vi "data_waypoint_ref.vi"() -> ()   [LabVIEW 2019] (continued)
"Y"=530152.5967771014}, {"X"=175289.23222510127, "Y"=530152.6409434144}, {"X"=175289.26360565764, "Y"=530152.6851751207}, {"X"=175289.29417483156, "Y"=530152.7294092241}, {"X"=175289.32498934455, "Y"=530152.7727347375}, {"X"=175289.35533826269, "Y"=530152.8164722754}, {"X"=175289.385890799, "Y"=530152.8604711375}, {"X"=175289.41661120942, "Y"=530152.904625996}, {"X"=175289.4478910891, "Y"=530152.9495616502}, {"X"=175289.47917020373, "Y"=530152.9951376967}, {"X"=175289.5106185431, "Y"=530153.0407265619}, {"X"=175289.54200313758, "Y"=530153.08602594}, {"X"=175289.5739645148, "Y"=530153.130472353}, {"X"=175289.60522496788, "Y"=530153.1748287205}, {"X"=175289.6366590831, "Y"=530153.2192023303}, {"X"=175289.6678968938, "Y"=530153.2639904988}, {"X"=175289.69931618578, "Y"=530153.3099423731}, {"X"=175289.73108270628, "Y"=530153.3561928844}, {"X"=175289.76287250203, "Y"=530153.402526566}, {"X"=175289.7944634813, "Y"=530153.4493247548}, {"X"=175289.82722049116, "Y"=530153.4953348278}, {"X"=175289.8601326513, "Y"=530153.5407928433}, {"X"=175289.89234136775, "Y"=530153.5862074348}, {"X"=175289.9231350958, "Y"=530153.6320945667}, {"X"=175289.95472487184, "Y"=530153.6784854437}, {"X"=175289.98763897427, "Y"=530153.7249001521}, {"X"=175290.0213877559, "Y"=530153.7711048503}, {"X"=175290.05441688612, "Y"=530153.8180774795}, {"X"=175290.0870279125, "Y"=530153.865045794}, {"X"=175290.1190894426, "Y"=530153.9119114052}, {"X"=175290.15082290868, "Y"=530153.9583695601}, {"X"=175290.18253651966, "Y"=530154.004402696}, {"X"=175290.215824471, "Y"=530154.0499339624}, {"X"=175290.24876343764, "Y"=530154.0957714727}, {"X"=175290.28090772417, "Y"=530154.1421662602}, {"X"=175290.31260737777, "Y"=530154.1888720124}, {"X"=175290.34510314872, "Y"=530154.2349083878}, {"X"=175290.37745346018, "Y"=530154.2805800489}, {"X"=175290.40967781737, "Y"=530154.3255950455}, {"X"=175290.4415173953, "Y"=530154.3698930992}, {"X"=175290.47334424395, "Y"=530154.4146795312}, {"X"=175290.50540644318, "Y"=530154.4602743543}, {"X"=175290.5380738031, "Y"=530154.5068251977}, {"X"=175290.57155401353, "Y"=530154.5544701797}, {"X"=175290.60687618723, "Y"=530154.6022528902}, {"X"=175290.64227715097, "Y"=530154.6503194917}, {"X"=175290.6771000642, "Y"=530154.6985121064}, {"X"=175290.71074572636, "Y"=530154.7463930005}, {"X"=175290.74366782108, "Y"=530154.7937166628}, {"X"=175290.77674741115, "Y"=530154.8397823889}, {"X"=175290.8104922183, "Y"=530154.8852446075}, {"X"=175290.84345047412, "Y"=530154.9319166768}, {"X"=175290.8771305831, "Y"=530154.9791648488}, {"X"=175290.91168912026, "Y"=530155.0269198505}, {"X"=175290.94661003543, "Y"=530155.0750045214}, {"X"=175290.981122192, "Y"=530155.1229516666}, {"X"=175291.01579159318, "Y"=530155.1701547412}, {"X"=175291.04955919375, "Y"=530155.2164370784}, {"X"=175291.08231414267, "Y"=530155.262653598}, {"X"=175291.11492730505, "Y"=530155.3085508951}, {"X"=175291.14872001382, "Y"=530155.3537377286}, {"X"=175291.182644366, "Y"=530155.3991095183}, {"X"=175291.21636701853, "Y"=530155.4442699214}, {"X"=175291.24936465317, "Y"=530155.4895811882}, {"X"=175291.28248111415, "Y"=530155.5349365}, {"X"=175291.31537208255, "Y"=530155.580122668}, {"X"=175291.348325878, "Y"=530155.6252864538}, {"X"=175291.38153227052, "Y"=530155.6705005467}, {"X"=175291.41516056712, "Y"=530155.7158055122}, {"X"=175291.44858402072, "Y"=530155.7616338248}, {"X"=175291.48274548614, "Y"=530155.8069127973}, {"X"=175291.51713847913, "Y"=530155.8517049672}, {"X"=175291.55134679007, "Y"=530155.8960504106}, {"X"=175291.58456519523, "Y"=530155.9396351947}, {"X"=175291.61696642355, "Y"=530155.9821591497}, {"X"=175291.6479902135, "Y"=530156.023771541}, {"X"=175291.6785537982, "Y"=530156.0649235916}, {"X"=175291.70969666803, "Y"=530156.1063669323}, {"X"=175291.7420121854, "Y"=530156.1480631868}, {"X"=175291.77421945485, "Y"=530156.1905977037}, {"X"=175291.80641845273, "Y"=530156.2342298953}, {"X"=175291.83880961206, "Y"=530156.2778426528}, {"X"=175291.8714862793, "Y"=530156.3212525729}, {"X"=175291.903615614, "Y"=530156.3652911794}, {"X"=175291.9363788722, "Y"=530156.4089272545}, {"X"=175291.9693198524, "Y"=530156.4530544727}, {"X"=175292.00263982284, "Y"=530156.4980373809}, {"X"=175292.03573972572, "Y"=530156.5440875158}, {"X"=175292.06968311957, "Y"=530156.5908099515}, {"X"=175292.10416577995, "Y"=530156.6374730819}, {"X"=175292.13854745447, "Y"=530156.6838335177}, {"X"=175292.1720661163, "Y"=530156.7301088271}, {"X"=175292.2050774269, "Y"=530156.7758551223}, {"X"=175292.23774666685, "Y"=530156.8212483841}, {"X"=175292.2703950841, "Y"=530156.8658914415}, {"X"=175292.30284617713, "Y"=530156.9103042324}, {"X"=175292.33573019976, "Y"=530156.9552418168}, {"X"=175292.3690841089, "Y"=530157.0006197365}, {"X"=175292.40287209605, "Y"=530157.0463115734}, {"X"=175292.43625491866, "Y"=530157.0924818472}, {"X"=175292.46991898818, "Y"=530157.1379065764}, {"X"=175292.50292587615, "Y"=530157.1830557807}, {"X"=175292.53606117488, "Y"=530157.2272967426}, {"X"=175292.56777705185, "Y"=530157.2717072674}, {"X"=175292.59928240773, "Y"=530157.317118397}, {"X"=175292.63191829307, "Y"=530157.3626160842}, {"X"=175292.66587593383, "Y"=530157.4075682566}, {"X"=175292.69985293486, "Y"=530157.4527767475}, {"X"=175292.73331970134, "Y"=530157.49827975}, {"X"=175292.76675738787, "Y"=530157.5444332153}, {"X"=175292.8009040642, "Y"=530157.5910063332}, {"X"=175292.8354354053, "Y"=530157.637958995}, {"X"=175292.87064782495, "Y"=530157.6854778919}, {"X"=175292.90666329346, "Y"=530157.7325748918}, {"X"=175292.94218916725, "Y"=530157.7803559012}, {"X"=175292.97651543948, "Y"=530157.8283546561}, {"X"=175293.01087843996, "Y"=530157.8758927135}, {"X"=175293.04497236086, "Y"=530157.9235003758}, {"X"=175293.07881658027, "Y"=530157.9705383087}, {"X"=175293.11260566092, "Y"=530158.0172023829}, {"X"=175293.14703717566, "Y"=530158.0636470264}, {"X"=175293.1813700373, "Y"=530158.1105791891}, {"X"=175293.21539555187, "Y"=530158.1584179054}, {"X"=175293.2495375595, "Y"=530158.205812335}, {"X"=175293.28470608912, "Y"=530158.252269229}, {"X"=175293.3199063943, "Y"=530158.2983886322}, {"X"=175293.35488698122, "Y"=530158.3438949328}, {"X"=175293.3886446154, "Y"=530158.389809945}, {"X"=175293.4223983855, "Y"=530158.4359169754}, {"X"=175293.45635716093, "Y"=530158.4824551338}, {"X"=175293.49104767398, "Y"=530158.5290177691}, {"X"=175293.52591940033, "Y"=530158.5751547926}, {"X"=175293.56061870293, "Y"=530158.6210958796}, {"X"=175293.59411550115, "Y"=530158.6668718222}, {"X"=175293.6271809516, "Y"=530158.7120597042}, {"X"=175293.65945930034, "Y"=530158.7576716585}, {"X"=175293.69267942, "Y"=530158.8030433188}, {"X"=175293.72706808845, "Y"=530158.8484792291}, {"X"=175293.76185547217, "Y"=530158.895451116}, {"X"=175293.7965144529, "Y"=530158.9433356876}, {"X"=175293.83203452808, "Y"=530158.9915551107}, {"X"=175293.86796527763, "Y"=530159.0399619979}, {"X"=175293.90361325, "Y"=530159.0885983519}, {"X"=175293.93887625565, "Y"=530159.1373534874}, {"X"=175293.97487363513, "Y"=530159.1852274456}, {"X"=175294.01073365632, "Y"=530159.2333814944}, {"X"=175294.04643691002, "Y"=530159.2821408798}, {"X"=175294.0818756446, "Y"=530159.3307123703}, {"X"=175294.11788264144, "Y"=530159.3791445598}, {"X"=175294.15405635608, "Y"=530159.4270401951}, {"X"=175294.19031250803, "Y"=530159.474657012}, {"X"=175294.2255617339, "Y"=530159.5217474012}, {"X"=175294.25969315338, "Y"=530159.5685591893}, {"X"=175294.29275883175, "Y"=530159.6156260639}, {"X"=175294.32651326683, "Y"=530159.6616609548}, {"X"=175294.3607518941, "Y"=530159.7075834295}, {"X"=175294.3953102612, "Y"=530159.754094294}, {"X"=175294.4301660572, "Y"=530159.800839571}, {"X"=175294.46538930168, "Y"=530159.8478312608}, {"X"=175294.5005892464, "Y"=530159.8944334593}, {"X"=175294.5360717114, "Y"=530159.9401191891}, {"X"=175294.57088286872, "Y"=530159.9855471951}, {"X"=175294.60512637242, "Y"=530160.0307227217}, {"X"=175294.63868134032, "Y"=530160.0764041571}, {"X"=175294.67373468378, "Y"=530160.1216560913}, {"X"=175294.7093190078, "Y"=530160.167040749}, {"X"=175294.74458629126, "Y"=530160.2136494077}, {"X"=175294.7794420138, "Y"=530160.2609707027}, {"X"=175294.81483305173, "Y"=530160.3092915086}, {"X"=175294.85090509735, "Y"=530160.3593561125}, {"X"=175294.88806120938, "Y"=530160.4102709948}, {"X"=175294.92585483048, "Y"=530160.4622982909}, {"X"=175294.96463635506, "Y"=530160.5147089018}, {"X"=175295.00314084318, "Y"=530160.5674932406}, {"X"=175295.04201721685, "Y"=530160.6190278914}, {"X"=175295.08002002342, "Y"=530160.6696039869}, {"X"=175295.1164572531, "Y"=530160.7191503169}, {"X"=175295.15120238528, "Y"=530160.7677160925}, {"X"=175295.18513989958, "Y"=530160.8154596288}, {"X"=175295.21911985, "Y"=530160.8622751979}, {"X"=175295.25361585215, "Y"=530160.908367834}, {"X"=175295.2882631498, "Y"=530160.9541026478}, {"X"=175295.3227068247, "Y"=530160.9995739195}, {"X"=175295.35650395526, "Y"=530161.0453733961}, {"X"=175295.39054459677, "Y"=530161.090246534}, {"X"=175295.4242712038, "Y"=530161.1346622286}, {"X"=175295.45741238436, "Y"=530161.1797045011}, {"X"=175295.49052893237, "Y"=530161.2251053321}, {"X"=175295.52422381577, "Y"=530161.2716753556}, {"X"=175295.5584969615, "Y"=530161.3190916035}, {"X"=175295.59356381797, "Y"=530161.3671225884}, {"X"=175295.62898613833, "Y"=530161.4158406355}, {"X"=175295.66490363725, "Y"=530161.4645672088}, {"X"=175295.70087106727, "Y"=530161.5140039441}, {"X"=175295.7368334574, "Y"=530161.563833585}, {"X"=175295.77286787695, "Y"=530161.6140581218}, {"X"=175295.80940447663, "Y"=530161.6645608615}, {"X"=175295.84631290415, "Y"=530161.7143954771}, {"X"=175295.88293148752, "Y"=530161.7641654665}, {"X"=175295.91866648968, "Y"=530161.8137837979}, {"X"=175295.95399056026, "Y"=530161.862829545}, {"X"=175295.9882959008, "Y"=530161.9112501208}, {"X"=175296.021704602, "Y"=530161.9589974427}, {"X"=175296.05467506434, "Y"=530162.0062210971}, {"X"=175296.08883693878, "Y"=530162.0522559017}, {"X"=175296.12335942886, "Y"=530162.0980232735}, {"X"=175296.15767913012, "Y"=530162.1438101135}, {"X"=175296.19184323237, "Y"=530162.18969841}, {"X"=175296.22616491732, "Y"=530162.2364574812}, {"X"=175296.26090724123, "Y"=530162.2837780067}, {"X"=175296.29650390253, "Y"=530162.3312458408}, {"X"=175296.33225156722, "Y"=530162.3800550482}, {"X"=175296.36839006183, "Y"=530162.4298308986}, {"X"=175296.40405752033, "Y"=530162.4808744899}, {"X"=175296.4404195736, "Y"=530162.5316652008}, {"X"=175296.4771856306, "Y"=530162.5818831403}, {"X"=175296.5143190418, "Y"=530162.6314185419}, {"X"=175296.55121999886, "Y"=530162.6796261277}, {"X"=175296.58696759774, "Y"=530162.7272156009}, {"X"=175296.62106253332, "Y"=530162.7745791067}, {"X"=175296.65513370547, "Y"=530162.8216951848}, {"X"=175296.6894842066, "Y"=530162.8689147633}, {"X"=175296.7245051825, "Y"=530162.9161112749}, {"X"=175296.7594826378, "Y"=530162.9641680548}, {"X"=175296.7949428259, "Y"=530163.0125164114}, {"X"=175296.83066872833, "Y"=530163.0611569866}, {"X"=175296.8668875833, "Y"=530163.1102511483}, {"X"=175296.90347265196, "Y"=530163.1594751914}, {"X"=175296.94033878695, "Y"=530163.2096906174}, {"X"=175296.97742890092, "Y"=530163.2601628694}, {"X"=175297.0145870955, "Y"=530163.3102930847}, {"X"=175297.0517672564, "Y"=530163.3603633035}, {"X"=175297.0892145761, "Y"=530163.4100154234}, {"X"=175297.1260384531, "Y"=530163.4594196689}, {"X"=175297.16179432158, "Y"=530163.5083098755}, {"X"=175297.1968335202, "Y"=530163.5568792308}, {"X"=175297.2321241116, "Y"=530163.6047908057}, {"X"=175297.26783519427, "Y"=530163.6517155846}, {"X"=175297.3031716078, "Y"=530163.6989466816}, {"X"=175297.3376430369, "Y"=530163.7460238435}, {"X"=175297.37241788793, "Y"=530163.7935651409}, {"X"=175297.40764496886, "Y"=530163.8421672372}, {"X"=175297.44412403886, "Y"=530163.8908943782}, {"X"=175297.4814756149, "Y"=530163.9405212577}, {"X"=175297.51936847973, "Y"=530163.9910710508}, {"X"=175297.5573672983, "Y"=530164.0433064074}, {"X"=175297.595877763, "Y"=530164.0960252604}, {"X"=175297.63482324645, "Y"=530164.1484764633}, {"X"=175297.67408375622, "Y"=530164.201420622}, {"X"=175297.71312810254, "Y"=530164.2540568792}, {"X"=175297.7516670672, "Y"=530164.3059288258}, {"X"=175297.78913671337, "Y"=530164.3565442422}, {"X"=175297.82573620637, "Y"=530164.4067560205}, {"X"=175297.8615577048, "Y"=530164.4559778853}, {"X"=175297.8972371134, "Y"=530164.5047762007}, {"X"=175297.93302551022, "Y"=530164.553887177}, {"X"=175297.96961301554, "Y"=530164.6033398478}, {"X"=175298.00658313325, "Y"=530164.653376285}, {"X"=175298.04413234367, "Y"=530164.7030403184}, {"X"=175298.08174063195, "Y"=530164.7529128302}, {"X"=175298.11949670635, "Y"=530164.8033376161}, {"X"=175298.15754264174, "Y"=530164.8535340244}, {"X"=175298.19573262517, "Y"=530164.9039153553}, {"X"=175298.2333517534, "Y"=530164.9547600736}, {"X"=175298.2709253971, "Y"=530165.0063984748}, {"X"=175298.30921058325, "Y"=530165.0575242384}, {"X"=175298.34725989297, "Y"=530165.108563021}, {"X"=175298.3849848592, "Y"=530165.160152141}, {"X"=175298.42313040857, "Y"=530165.2113859762}, {"X"=175298.46161175598, "Y"=530165.2629473361}, {"X"=175298.5006422235, "Y"=530165.3141863251}, {"X"=175298.53957860355, "Y"=530165.3662590976}, {"X"=175298.57924604914, "Y"=530165.4196282434}, {"X"=175298.61979824462, "Y"=530165.4744453614}, {"X"=175298.66179051698, "Y"=530165.5306877274}, {"X"=175298.70499840498, "Y"=530165.5885357952}, {"X"=175298.74955290352, "Y"=530165.6482533285}, {"X"=175298.79480152024, "Y"=530165.7087545921}, {"X"=175298.83997422215, "Y"=530165.7702460737}, {"X"=175298.8847225618, "Y"=530165.8314136203}, {"X"=175298.9291021474, "Y"=530165.8912926009}, {"X"=175298.97281817885, "Y"=530165.9496397171}, {"X"=175299.01543963805, "Y"=530166.0068768775}, {"X"=175299.05688362545, "Y"=530166.0634271845}, {"X"=175299.09825262203, "Y"=530166.1191808339}, {"X"=175299.13975714424, "Y"=530166.173434664}, {"X"=175299.18070865513, "Y"=530166.2269953544}, {"X"=175299.22062828136, "Y"=530166.2793770946}, {"X"=175299.25974002617, "Y"=530166.3308455878}, {"X"=175299.297952328, "Y"=530166.3812912287}, {"X"=175299.33612488734, "Y"=530166.4305771838}, {"X"=175299.37402761978, "Y"=530166.4784788326}, {"X"=175299.41189246927, "Y"=530166.5255504185}, {"X"=175299.44854593184, "Y"=530166.5730484385}, {"X"=175299.48464680242, "Y"=530166.620295045}, {"X"=175299.5206186963, "Y"=530166.667360014}, {"X"=175299.5570817157, "Y"=530166.7139596118}, {"X"=175299.59393444148, "Y"=530166.760246189}, {"X"=175299.63101704643, "Y"=530166.8075875615}, {"X"=175299.66873832993, "Y"=530166.8558371342}, {"X"=175299.70755977381, "Y"=530166.9049891003}, {"X"=175299.74702618556, "Y"=530166.954779551}, {"X"=175299.78702946118, "Y"=530167.0048947148}, {"X"=175299.8269780119, "Y"=530167.0550766316}, {"X"=175299.86691015412, "Y"=530167.1045016735}, {"X"=175299.9056200963, "Y"=530167.1539902581}, {"X"=175299.94444108658, "Y"=530167.202690514}, {"X"=175299.9832469312, "Y"=530167.2507615263}, {"X"=175300.02239172766, "Y"=530167.2984286564}, {"X"=175300.06160983795, "Y"=530167.3454263278}, {"X"=175300.10023907598, "Y"=530167.3924845605}, {"X"=175300.13795698716, "Y"=530167.4389938845}, {"X"=175300.17463229306, "Y"=530167.4854940797}, {"X"=175300.21027157555, "Y"=530167.53151233}, {"X"=175300.2456148467, "Y"=530167.5762784209}, {"X"=175300.28083256615, "Y"=530167.6208229107}, {"X"=175300.31683014592, "Y"=530167.6648911891}, {"X"=175300.35295156413, "Y"=530167.7092010507}, {"X"=175300.38885968522, "Y"=530167.754471571}, {"X"=175300.42531408952, "Y"=530167.7996572366}, {"X"=175300.4626722015, "Y"=530167.8446127126}, {"X"=175300.49978768127, "Y"=530167.8895922136}, {"X"=175300.5366776678, "Y"=530167.9350018955}, {"X"=175300.57296706524, "Y"=530167.9810026871}, {"X"=175300.60997343756, "Y"=530168.02653078}, {"X"=175300.64725950157, "Y"=530168.0722844577}, {"X"=175300.6848355032, "Y"=530168.1178341768}, {"X"=175300.72194708392, "Y"=530168.1629945957}, {"X"=175300.75843372697, "Y"=530168.2077007085}, {"X"=175300.79459920572, "Y"=530168.2516353095}, {"X"=175300.8309390622, "Y"=530168.2958279934}, {"X"=175300.86721646803, "Y"=530168.3407689049}, {"X"=175300.9041467231, "Y"=530168.3860186503}, {"X"=175300.94086441226, "Y"=530168.431876116}, {"X"=175300.97748970473, "Y"=530168.4773398549}, {"X"=175301.01311529457, "Y"=530168.5226245311}, {"X"=175301.04880451673, "Y"=530168.5675605212}, {"X"=175301.08470138145, "Y"=530168.6111218947}, {"X"=175301.11998015357, "Y"=530168.6544464744}, {"X"=175301.1544579749, "Y"=530168.6983050416}, {"X"=175301.1899404005, "Y"=530168.7422039253}, {"X"=175301.2262133977, "Y"=530168.787153732}, {"X"=175301.26329977365, "Y"=530168.8327792599}, {"X"=175301.30040072044, "Y"=530168.8794402435}, {"X"=175301.33783310797, "Y"=530168.9261524099}, {"X"=175301.37482062684, "Y"=530168.9724974196}, {"X"=175301.41083388752, "Y"=530169.0185789398}, {"X"=175301.44611475465, "Y"=530169.0635150287}, {"X"=175301.48104166967, "Y"=530169.107673044}, {"X"=175301.515584441, "Y"=530169.1522306317}, {"X"=175301.5505684368, "Y"=530169.1965216612}, {"X"=175301.58586430468, "Y"=530169.2408384063}, {"X"=175301.621437572, "Y"=530169.2849046132}, {"X"=175301.65624651004, "Y"=530169.3287078214}, {"X"=175301.69067446323, "Y"=530169.3715787638}, {"X"=175301.72433513994, "Y"=530169.4131889531}, {"X"=175301.7572057744, "Y"=530169.4545273413}, {"X"=175301.7897156011, "Y"=530169.4957669071}, {"X"=175301.82262842666, "Y"=530169.5363948606}, {"X"=175301.85541520052, "Y"=530169.5775315022}, {"X"=175301.88877971005, "Y"=530169.6193356836}, {"X"=175301.92198627733, "Y"=530169.6622479695}, {"X"=175301.9549979493, "Y"=530169.7066524813}, {"X"=175301.98874946675, "Y"=530169.7514277223}, {"X"=175302.02408231725, "Y"=530169.7962715428}, {"X"=175302.05988879167, "Y"=530169.84162117}, {"X"=175302.09521931363, "Y"=530169.886875645}, {"X"=175302.12915909418, "Y"=530169.9324128029}, {"X"=175302.16313239714, "Y"=530169.9770042623}, {"X"=175302.19741865405, "Y"=530170.0198878336}, {"X"=175302.23161996814, "Y"=530170.0622022983}, {"X"=175302.2647214002, "Y"=530170.1043091388}, {"X"=175302.29732747353, "Y"=530170.1466471837}, {"X"=175302.32942471874, "Y"=530170.1900533064}, {"X"=175302.36214685687, "Y"=530170.2339004164}, {"X"=175302.39546431036, "Y"=530170.2777679664}, {"X"=175302.42970125427, "Y"=530170.3213508952}, {"X"=175302.46371953157, "Y"=530170.3649755353}, {"X"=175302.4970483943, "Y"=530170.409108309}, {"X"=175302.53014454423, "Y"=530170.452725684}, {"X"=175302.56359763598, "Y"=530170.4957338027}, {"X"=175302.59699459223, "Y"=530170.5389285439}, {"X"=175302.63076028306, "Y"=530170.5819079936}, {"X"=175302.6641188947, "Y"=530170.625916373}, {"X"=175302.6977430426, "Y"=530170.6704567027}, {"X"=175302.7314268824, "Y"=530170.7154141635}, {"X"=175302.76559054904, "Y"=530170.7605799701}, {"X"=175302.80000400502, "Y"=530170.8048449432}, {"X"=175302.83450216462, "Y"=530170.8486979064}, {"X"=175302.868423361, "Y"=530170.8930431358}, {"X"=175302.9020594507, "Y"=530170.9368298354}, {"X"=175302.93501567593, "Y"=530170.9804587241}, {"X"=175302.96820232505, "Y"=530171.0238283353}, {"X"=175303.0014239085, "Y"=530171.0667294834}, {"X"=175303.03441731303, "Y"=530171.1100519415}, {"X"=175303.06691230068, "Y"=530171.153469102}, {"X"=175303.09917383848, "Y"=530171.1964219182}, {"X"=175303.13118923537, "Y"=530171.2397117508}, {"X"=175303.1637000194, "Y"=530171.2824795955}, {"X"=175303.19595648517, "Y"=530171.3261138815}, {"X"=175303.22875163666, "Y"=530171.3703914051}, {"X"=175303.26162110508, "Y"=530171.4149395159}, {"X"=175303.2943639709, "Y"=530171.4604080732}, {"X"=175303.3270933593, "Y"=530171.5061119605}, {"X"=175303.36078521397, "Y"=530171.5507863855}, {"X"=175303.39476642053, "Y"=530171.5950592977}, {"X"=175303.42826067653, "Y"=530171.6391105651}, {"X"=175303.46060070378, "Y"=530171.683447147}, {"X"=175303.4932010295, "Y"=530171.7277418941}, {"X"=175303.5264554045, "Y"=530171.7715508118}, {"X"=175303.56027406864, "Y"=530171.815673263}, {"X"=175303.59372100336, "Y"=530171.8604982444}, {"X"=175303.62725594908, "Y"=530171.9051320691}, {"X"=175303.66013932397, "Y"=530171.9501906737}, {"X"=175303.69312924595, "Y"=530171.9947339906}, {"X"=175303.72571887134, "Y"=530172.0390054631}, {"X"=175303.75856571438, "Y"=530172.0833916041}, {"X"=175303.7914979888, "Y"=530172.1276121215}, {"X"=175303.82426099747, "Y"=530172.1724058269}, {"X"=175303.85658823774, "Y"=530172.2175126894}, {"X"=175303.8893403862, "Y"=530172.2622276273}, {"X"=175303.9219982045, "Y"=530172.3070960032}, {"X"=175303.95487855875, "Y"=530172.3514321018}, {"X"=175303.98756941865, "Y"=530172.395190523}, {"X"=175304.0198873744, "Y"=530172.4383540505}, {"X"=175304.05146210626, "Y"=530172.4803022576}, {"X"=175304.08243248635, "Y"=530172.5218682386}, {"X"=175304.11302771606, "Y"=530172.5638781629}, {"X"=175304.14440576072, "Y"=530172.6058125234}, {"X"=175304.17647083785, "Y"=530172.6485317448}, {"X"=175304.2092485257, "Y"=530172.6916983553}, {"X"=175304.2421544904, "Y"=530172.7351098659}, {"X"=175304.27474581596, "Y"=530172.7793591394}, {"X"=175304.30713692037, "Y"=530172.8241972291}, {"X"=175304.33966600779, "Y"=530172.8692668731}, {"X"=175304.3725380399, "Y"=530172.9146862191}, {"X"=175304.40615073708, "Y"=530172.9595551069}, {"X"=175304.43922888403, "Y"=530173.0045820643}, {"X"=175304.47193721798, "Y"=530173.0500607167}, {"X"=175304.50408048517, "Y"=530173.095561017}, {"X"=175304.53664703757, "Y"=530173.1407204481}, {"X"=175304.57019344828, "Y"=530173.1850401526}, {"X"=175304.60417604624, "Y"=530173.229188761}, {"X"=175304.63733822326, "Y"=530173.274475177}, {"X"=175304.67012666404, "Y"=530173.3200845581}, {"X"=175304.70293440312, "Y"=530173.3656295104}, {"X"=175304.73601901694, "Y"=530173.4107485677}, {"X"=175304.7688052838, "Y"=530173.4550216836}, {"X"=175304.80180875398, "Y"=530173.4984595454}, {"X"=175304.83439683876, "Y"=530173.5410129662}, {"X"=175304.86641084577, "Y"=530173.5832384543}, {"X"=175304.89706473134, "Y"=530173.6259163404}, {"X"=175304.92851563115, "Y"=530173.6676274072}, {"X"=175304.96001501603, "Y"=530173.7089609802}, {"X"=175304.9911972434, "Y"=530173.7511778257}, {"X"=175305.0218017102, "Y"=530173.7939191228}, {"X"=175305.0528701443, "Y"=530173.8368965593}, {"X"=175305.0845467455, "Y"=530173.8803494384}, {"X"=175305.11676661787, "Y"=530173.9241980441}, {"X"=175305.1485606208, "Y"=530173.9687116023}, {"X"=175305.1810053819, "Y"=530174.0134252321}, {"X"=175305.21403351048, "Y"=530174.0580150564}, {"X"=175305.24728412752, "Y"=530174.1035575917}, {"X"=175305.28061614945, "Y"=530174.1499689076}, {"X"=175305.31471056672, "Y"=530174.1962902915}, {"X"=175305.3486507356, "Y"=530174.243170392}, {"X"=175305.3823800229, "Y"=530174.2900289173}, {"X"=175305.4154933949, "Y"=530174.3367893738}, {"X"=175305.4486278848, "Y"=530174.3826019497}, {"X"=175305.48151879795, "Y"=530174.4275195878}, {"X"=175305.5138967311, "Y"=530174.4724010066}, {"X"=175305.54595081756, "Y"=530174.517701799}, {"X"=175305.57926572644, "Y"=530174.562519407}, {"X"=175305.61313334163, "Y"=530174.6076283868}, {"X"=175305.64742550213, "Y"=530174.6531223445}, {"X"=175305.68094282097, "Y"=530174.6995930464}, {"X"=175305.7142195681, "Y"=530174.7464862061}, {"X"=175305.74732664338, "Y"=530174.7932144965}, {"X"=175305.78057287785, "Y"=530174.8402742251}, {"X"=175305.8133739154, "Y"=530174.8877536852}, {"X"=175305.84608374408, "Y"=530174.9352422942}, {"X"=175305.8802467283, "Y"=530174.9825878779}, {"X"=175305.91585264518, "Y"=530175.02962732}, {"X"=175305.95117603574, "Y"=530175.0772802396}, {"X"=175305.98675250847, "Y"=530175.1248480605}, {"X"=175306.0226269634, "Y"=530175.1719366532}, {"X"=175306.05766248834, "Y"=530175.219295199}, {"X"=175306.09146300732, "Y"=530175.2665819227}, {"X"=175306.1256061778, "Y"=530175.3138176922}, {"X"=175306.15987830423, "Y"=530175.3612284362}, {"X"=175306.19375731278, "Y"=530175.4089977182}, {"X"=175306.2272617157, "Y"=530175.4570955143}, {"X"=175306.26149442443, "Y"=530175.5043554353}, {"X"=175306.29601557076, "Y"=530175.5512049651}, {"X"=175306.33110052024, "Y"=530175.5979052205}, {"X"=175306.3664420601, "Y"=530175.6445070498}, {"X"=175306.40137430347, "Y"=530175.6922876495}, {"X"=175306.43611313298, "Y"=530175.7405627077}, {"X"=175306.47135692826, "Y"=530175.7888606924}, {"X"=175306.50683563814, "Y"=530175.836619701}, {"X"=175306.5427093849, "Y"=530175.8837704501}, {"X"=175306.57804036967, "Y"=530175.9312979346}, {"X"=175306.61314321528, "Y"=530175.9786596134}, {"X"=175306.64723720393, "Y"=530176.0260398111}, {"X"=175306.68197792507, "Y"=530176.0728576195}, {"X"=175306.71729545467, "Y"=530176.1191287831}, {"X"=175306.75288187485, "Y"=530176.1655689615}, {"X"=175306.78805515857, "Y"=530176.2121868278}, {"X"=175306.82317604765, "Y"=530176.2593597791}, {"X"=175306.85816065417, "Y"=530176.3068771907}, {"X"=175306.89302999235, "Y"=530176.3543549852}, {"X"=175306.92829042548, "Y"=530176.4019892259}, {"X"=175306.96434128538, "Y"=530176.4494269079}, {"X"=175307.0002629, "Y"=530176.4974909314}, {"X"=175307.03651319438, "Y"=530176.5461732863}, {"X"=175307.07280654478, "Y"=530176.5944370972}, {"X"=175307.10929617652, "Y"=530176.6425793526}, {"X"=175307.1459389947, "Y"=530176.6904026284}, {"X"=175307.1830941412, "Y"=530176.738340926}, {"X"=175307.2198662148, "Y"=530176.7870406077}, {"X"=175307.25608431565, "Y"=530176.836519937}, {"X"=175307.2923623031, "Y"=530176.8870823126}, {"X"=175307.32952882035, "Y"=530176.9370727075}, {"X"=175307.36630468437, "Y"=530176.9870564856}, {"X"=175307.40306440124, "Y"=530177.0369715019}, {"X"=175307.43982546963, "Y"=530177.0867444496}, {"X"=175307.47700678377, "Y"=530177.1363463515}, {"X"=175307.51413816065, "Y"=530177.1855366402}, {"X"=175307.55166098283, "Y"=530177.2347013578}, {"X"=175307.58907466935, "Y"=530177.2841050166}, {"X"=175307.62627763985, "Y"=530177.3341430286}, {"X"=175307.66311196302, "Y"=530177.3850267321}, {"X"=175307.7005225817, "Y"=530177.4357899772}, {"X"=175307.73824461747, "Y"=530177.486425782}, {"X"=175307.77605915256, "Y"=530177.5362899586}, {"X"=175307.81286147056, "Y"=530177.5865344778}, {"X"=175307.84951953805, "Y"=530177.6365241562}, {"X"=175307.88651088442, "Y"=530177.6859901074}, {"X"=175307.92401568915, "Y"=530177.7353546531}, {"X"=175307.9616221725, "Y"=530177.7846556385}, {"X"=175307.99953877402, "Y"=530177.8345883267}, {"X"=175308.03749193915, "Y"=530177.884904919}, {"X"=175308.07523145544, "Y"=530177.9354618721}, {"X"=175308.11299889255, "Y"=530177.9858755714}, {"X"=175308.15146935455, "Y"=530178.0352905402}, {"X"=175308.1892898605, "Y"=530178.0844787983}, {"X"=175308.2265397046, "Y"=530178.1335943816}, {"X"=175308.26328121778, "Y"=530178.1833474154}, {"X"=175308.30082930517, "Y"=530178.2326729915}, {"X"=175308.3391933072, "Y"=530178.2817331203}, {"X"=175308.37776592822, "Y"=530178.3309480151}, {"X"=175308.41586902775, "Y"=530178.3798457655}, {"X"=175308.45360439137, "Y"=530178.4289987606}, {"X"=175308.49054393347, "Y"=530178.4786213585}, {"X"=175308.52805617274, "Y"=530178.5275064252}, {"X"=175308.56581533956, "Y"=530178.5760211812}, {"X"=175308.60384613005, "Y"=530178.6241300373}, {"X"=175308.6412520306, "Y"=530178.6727002201}, {"X"=175308.67826697233, "Y"=530178.7214602334}, {"X"=175308.71486306612, "Y"=530178.7711648659}, {"X"=175308.75246034496, "Y"=530178.8215513228}, {"X"=175308.7912765256, "Y"=530178.872557922}, {"X"=175308.83084101314, "Y"=530178.9247021361}, {"X"=175308.8709113982, "Y"=530178.9771833654}, {"X"=175308.9109508622, "Y"=530179.0296935422}, {"X"=175308.95094127575, "Y"=530179.0814902235}, {"X"=175308.99123117467, "Y"=530179.1321184501}, {"X"=175309.03012990014, "Y"=530179.1819827599}, {"X"=175309.0674750189, "Y"=530179.2309682134}, {"X"=175309.1034754659, "Y"=530179.2796402158}, {"X"=175309.13934451604, "Y"=530179.327610065}, {"X"=175309.1753644265, "Y"=530179.3756738087}, {"X"=175309.21217135477, "Y"=530179.4232857344}, {"X"=175309.24893715564, "Y"=530179.4707690383}, {"X"=175309.28518585657, "Y"=530179.5189197841}, {"X"=175309.32090653412, "Y"=530179.5670399042}, {"X"=175309.35713197305, "Y"=530179.6151130308}, {"X"=175309.3934266228, "Y"=530179.6635266797}, {"X"=175309.42987620586, "Y"=530179.712513667}, {"X"=175309.46639058788, "Y"=530179.7624460628}, {"X"=175309.50371548356, "Y"=530179.8120852838}, {"X"=175309.5409782049, "Y"=530179.8619666371}, {"X"=175309.5787927472, "Y"=530179.9121404743}, {"X"=175309.61645778242, "Y"=530179.9635788811}, {"X"=175309.65459812188, "Y"=530180.0163932223}, {"X"=175309.69325909083, "Y"=530180.0694357668}, {"X"=175309.7317165625, "Y"=530180.122557711}, {"X"=175309.76908308847, "Y"=530180.1751967588}, {"X"=175309.80636802042, "Y"=530180.2269015467}, {"X"=175309.84373904276, "Y"=530180.2774640337}, {"X"=175309.88096197287, "Y"=530180.3267706002}, {"X"=175309.91734318458, "Y"=530180.3757034084}, {"X"=175309.9532567708, "Y"=530180.4237596989}, {"X"=175309.98798831712, "Y"=530180.472282293}, {"X"=175310.02238339974, "Y"=530180.5208502738}, {"X"=175310.0573020126, "Y"=530180.5694289177}, {"X"=175310.09330661935, "Y"=530180.6183128951}, {"X"=175310.12955154193, "Y"=530180.6672871724}, {"X"=175310.1658978246, "Y"=530180.7169914382}, {"X"=175310.20254698073, "Y"=530180.7669722736}, {"X"=175310.23967130386, "Y"=530180.817684213}, {"X"=175310.2773086728, "Y"=530180.8690550049}, {"X"=175310.3148211599, "Y"=530180.9201309427}, {"X"=175310.3511979726, "Y"=530180.9723744758}, {"X"=175310.38740139623, "Y"=530181.0252955357}, {"X"=175310.42416107788, "Y"=530181.0797110443}, {"X"=175310.4624049127, "Y"=530181.1348802013}, {"X"=175310.50164816767, "Y"=530181.1901351993}, {"X"=175310.54203527907, "Y"=530181.244894042}, {"X"=175310.58194975206, "Y"=530181.2991792613}, {"X"=175310.62001042886, "Y"=530181.3529172424}, {"X"=175310.65622358862, "Y"=530181.4049370685}, {"X"=175310.69123930926, "Y"=530181.4558061787}, {"X"=175310.72519802517, "Y"=530181.5047872087}, {"X"=175310.75874079563, "Y"=530181.5520969089}, {"X"=175310.79136085967, "Y"=530181.5980020331}, {"X"=175310.82360926468, "Y"=530181.6437328964}, {"X"=175310.85623968006, "Y"=530181.6907456301}, {"X"=175310.8897590421, "Y"=530181.7388267526}, {"X"=175310.9243145624, "Y"=530181.7880357637}, {"X"=175310.959343698, "Y"=530181.8383487933}, {"X"=175310.99435753067, "Y"=530181.8885797397}, {"X"=175311.0290962056, "Y"=530181.9392199271}, {"X"=175311.06388729028, "Y"=530181.990211786}, {"X"=175311.09868500763, "Y"=530182.0416486778}, {"X"=175311.13335366588, "Y"=530182.0931758506}, {"X"=175311.16810784728, "Y"=530182.1445684781}, {"X"=175311.20274703568, "Y"=530182.1960147172}, {"X"=175311.2379057422, "Y"=530182.2467135971}, {"X"=175311.27227776014, "Y"=530182.2976745092}, {"X"=175311.30606672564, "Y"=530182.3482675583}, {"X"=175311.3395601565, "Y"=530182.3986683643}, {"X"=175311.37393442274, "Y"=530182.448891213}, {"X"=175311.40852775157, "Y"=530182.4980068854}, {"X"=175311.44232597886, "Y"=530182.5478374333}, {"X"=175311.475157056, "Y"=530182.5983112288}, {"X"=175311.50801931764, "Y"=530182.6491478536}, {"X"=175311.54183613407, "Y"=530182.6998740053}, {"X"=175311.57663097818, "Y"=530182.7503397807}, {"X"=175311.61155363472, "Y"=530182.8014932929}, {"X"=175311.64626777923, "Y"=530182.8537284222}, {"X"=175311.68068305723, "Y"=530182.906743557}, {"X"=175311.7154702105, "Y"=530182.9591049955}, {"X"=175311.75001092287, "Y"=530183.0102019231}, {"X"=175311.78433634012, "Y"=530183.0606824049}, {"X"=175311.8183494312, "Y"=530183.1100850247}, {"X"=175311.8516716377, "Y"=530183.1588970209}, {"X"=175311.88408727964, "Y"=530183.2072721894}, {"X"=175311.91671428684, "Y"=530183.2552338662}, {"X"=175311.94992222873, "Y"=530183.3031472128}, {"X"=175311.98340970423, "Y"=530183.3515336459}, {"X"=175312.01677082642, "Y"=530183.4009259832}, {"X"=175312.0510007853, "Y"=530183.4505787942}, {"X"=175312.08557931965, "Y"=530183.5009863878}, {"X"=175312.12013653468, "Y"=530183.5522741646}, {"X"=175312.1542311072, "Y"=530183.6031737451}, {"X"=175312.1881540991, "Y"=530183.6538618514}, {"X"=175312.22243575216, "Y"=530183.7045222601}, {"X"=175312.25757506452, "Y"=530183.7549559459}, {"X"=175312.29278177244, "Y"=530183.8060153938}, {"X"=175312.32824544844, "Y"=530183.8574059312}, {"X"=175312.36394127307, "Y"=530183.9094206324}, {"X"=175312.4001556887, "Y"=530183.9609732128}, {"X"=175312.43641827087, "Y"=530184.0123380839}, {"X"=175312.4721263033, "Y"=530184.0636879449}, {"X"=175312.5069555313, "Y"=530184.1153023272}, {"X"=175312.54130807726, "Y"=530184.1674741576}, {"X"=175312.57628509818, "Y"=530184.2193444809}, {"X"=175312.61243834853, "Y"=530184.2708817059}, {"X"=175312.64919719583, "Y"=530184.3226235745}, {"X"=175312.68595615213, "Y"=530184.375303274}, {"X"=175312.72274589876, "Y"=530184.4288108387}, {"X"=175312.76002624852, "Y"=530184.4819762268}, {"X"=175312.79754509203, "Y"=530184.5349156114}, {"X"=175312.83499864914, "Y"=530184.5870438805}, {"X"=175312.8714617927, "Y"=530184.639437001}, {"X"=175312.90760069605, "Y"=530184.6915169893}, {"X"=175312.94404201457, "Y"=530184.7425184103}, {"X"=175312.98059682967, "Y"=530184.792660466}, {"X"=175313.01660241385, "Y"=530184.8418874011}, {"X"=175313.0520811022, "Y"=530184.891164725}, {"X"=175313.08734580636, "Y"=530184.9402695426}, {"X"=175313.12239439436, "Y"=530184.9893805474}, {"X"=175313.15734865, "Y"=530185.0386427735}, {"X"=175313.19286568387, "Y"=530185.0874072288}, {"X"=175313.22880935456, "Y"=530185.1363668718}, {"X"=175313.2649331918, "Y"=530185.1854447369}, {"X"=175313.30088473303, "Y"=530185.2346696118}, {"X"=175313.33722131583, "Y"=530185.2841008937}, {"X"=175313.37432573305, "Y"=530185.3331847425}, {"X"=175313.41198690207, "Y"=530185.3824289885}, {"X"=175313.449257545, "Y"=530185.4320095631}, {"X"=175313.48641791966, "Y"=530185.4820455073}, {"X"=175313.52345464373, "Y"=530185.5322027901}, {"X"=175313.56054014363, "Y"=530185.581779473}, {"X"=175313.59761448327, "Y"=530185.6311763932}, {"X"=175313.63479581906, "Y"=530185.6799115203}, {"X"=175313.67125340502, "Y"=530185.7286254782}, {"X"=175313.7071050316, "Y"=530185.7767130446}, {"X"=175313.74212418348, "Y"=530185.8236565841}, {"X"=175313.77722887165, "Y"=530185.8701692459}, {"X"=175313.8128344303, "Y"=530185.915917957}, {"X"=175313.8479152154, "Y"=530185.9618358053}, {"X"=175313.8821893614, "Y"=530186.0081600237}, {"X"=175313.9155590152, "Y"=530186.0544491778}, {"X"=175313.94968215242, "Y"=530186.1009303334}, {"X"=175313.98505024164, "Y"=530186.1469527704}, {"X"=175314.021090573, "Y"=530186.1929521351}, {"X"=175314.0570167525, "Y"=530186.2398907787}, {"X"=175314.0929765313, "Y"=530186.2871078982}, {"X"=175314.12863386451, "Y"=530186.3353935948}, {"X"=175314.16455866926, "Y"=530186.3845663889}, {"X"=175314.20138941368, "Y"=530186.4342648024}, {"X"=175314.2386463122, "Y"=530186.4848942381}, {"X"=175314.2759694681, "Y"=530186.5360639819}, {"X"=175314.31256280615, "Y"=530186.5878574002}, {"X"=175314.34945666775, "Y"=530186.638833074}, {"X"=175314.3865433375, "Y"=530186.6888093075}, {"X"=175314.42391436658, "Y"=530186.7372930504}, {"X"=175314.46051972595, "Y"=530186.7847590921}, {"X"=175314.49610486344, "Y"=530186.8319939679}, {"X"=175314.53065131142, "Y"=530186.8787435716}, {"X"=175314.56469552708, "Y"=530186.925797649}, {"X"=175314.5991626018, "Y"=530186.9729659047}, {"X"=175314.63475583828, "Y"=530187.0199443783}, {"X"=175314.6702479863, "Y"=530187.0677866219}, {"X"=175314.70570368378, "Y"=530187.1158842411}, {"X"=175314.74113296997, "Y"=530187.1637366577}, {"X"=175314.7767761707, "Y"=530187.2114375022}, {"X"=175314.8127982049, "Y"=530187.2590428923}, {"X"=175314.84901318164, "Y"=530187.3068952105}, {"X"=175314.88495516544, "Y"=530187.354989174}, {"X"=175314.92082059308, "Y"=530187.4035550535}, {"X"=175314.9563999271, "Y"=530187.4521262179}, {"X"=175314.99203503237, "Y"=530187.5000867952}, {"X"=175315.027573906, "Y"=530187.5481553137}, {"X"=175315.06366672198, "Y"=530187.5957349675}, {"X"=175315.09989612902, "Y"=530187.6433741514}, {"X"=175315.13577743215, "Y"=530187.6919177884}, {"X"=175315.17143027333, "Y"=530187.7407861799}, {"X"=175315.2078786093, "Y"=530187.7896733094}, {"X"=175315.24473079812, "Y"=530187.8379388351}, {"X"=175315.28113080456, "Y"=530187.8863588558}, {"X"=175315.3168192751, "Y"=530187.9346944091}, {"X"=175315.35221031535, "Y"=530187.9824947795}, {"X"=175315.3872724083, "Y"=530188.0301884642}, {"X"=175315.4232301929, "Y"=530188.0770360122}, {"X"=175315.45946732393, "Y"=530188.1242933825}, {"X"=175315.49556506728, "Y"=530188.172942929}, {"X"=175315.53165468454, "Y"=530188.2221396589}, {"X"=175315.5681028295, "Y"=530188.2712643011}, {"X"=175315.6050792257, "Y"=530188.319897936}, {"X"=175315.64205526988, "Y"=530188.3684117062}, {"X"=175315.67818000304, "Y"=530188.4163031384}, {"X"=175315.71349551325, "Y"=530188.4634256088}, {"X"=175315.7479487243, "Y"=530188.5107026764}, {"X"=175315.78355792633, "Y"=530188.5570928828}, {"X"=175315.8199135922, "Y"=530188.6030968745}, {"X"=175315.85587449878, "Y"=530188.6498034624}, {"X"=175315.890835794, "Y"=530188.6969602753}, {"X"=175315.92577562438, "Y"=530188.7449473259}, {"X"=175315.96154261148, "Y"=530188.7925767798}, {"X"=175315.99833612668, "Y"=530188.8407736705}, {"X"=175316.03534774587, "Y"=530188.8896380548}, {"X"=175316.07250852248, "Y"=530188.9386196402}, {"X"=175316.10918241073, "Y"=530188.9883018779}, {"X"=175316.14599503172, "Y"=530189.0375697273}, {"X"=175316.18267309142, "Y"=530189.0859634053}, {"X"=175316.21865495804, "Y"=530189.1340705757}, {"X"=175316.2542279634, "Y"=530189.1823032569}, {"X"=175316.28991713698, "Y"=530189.2311815331}, {"X"=175316.32575928187, "Y"=530189.2802680123}, {"X"=175316.36204323257, "Y"=530189.3298859186}, {"X"=175316.39863125872, "Y"=530189.3786882918}, {"X"=175316.43458270805, "Y"=530189.426994219}, {"X"=175316.4692830125, "Y"=530189.4751606653}, {"X"=175316.5038935927, "Y"=530189.5220388316}, {"X"=175316.5382121839, "Y"=530189.5681254207}, {"X"=175316.57219325224, "Y"=530189.6144993486}, {"X"=175316.60615941638, "Y"=530189.6612262579}, {"X"=175316.64103085897, "Y"=530189.7085542566}, {"X"=175316.67637426974, "Y"=530189.7564302428}, {"X"=175316.71164391257, "Y"=530189.8054218558}, {"X"=175316.74676780688, "Y"=530189.8548511842}, {"X"=175316.78219569896, "Y"=530189.9043395466}, {"X"=175316.8177323982, "Y"=530189.9537787547}, {"X"=175316.85369295246, "Y"=530190.0021701136}, {"X"=175316.8896444052, "Y"=530190.050779032}, {"X"=175316.92564777914, "Y"=530190.1001735788}, {"X"=175316.9620438199, "Y"=530190.1499565273}, {"X"=175316.99894420846, "Y"=530190.1998534118}, {"X"=175317.03558734115, "Y"=530190.2499219743}, {"X"=175317.07208662984, "Y"=530190.3004748595}, {"X"=175317.1083717217, "Y"=530190.3504823267}, {"X"=175317.1443335403, "Y"=530190.400203296}, {"X"=175317.18068957215, "Y"=530190.4502371901}, {"X"=175317.21824675493, "Y"=530190.4999789775}, {"X"=175317.25626110364, "Y"=530190.5500545918}, {"X"=175317.29395553737, "Y"=530190.6003819788}, {"X"=175317.3309519411, "Y"=530190.6512985411}, {"X"=175317.36805747618, "Y"=530190.7025765971}, {"X"=175317.40498688072, "Y"=530190.7539028961}, {"X"=175317.4429407785, "Y"=530190.8048066457}, {"X"=175317.48180363432, "Y"=530190.8554568817}, {"X"=175317.52073454688, "Y"=530190.9072578424}, {"X"=175317.55972893158, "Y"=530190.9592550602}, {"X"=175317.59894806604, "Y"=530191.0108720445}, {"X"=175317.6377611856, "Y"=530191.0620784669}, {"X"=175317.67635760055, "Y"=530191.1127916438}, {"X"=175317.7140501114, "Y"=530191.1633687577}, {"X"=175317.75095119307, "Y"=530191.2141035862}, {"X"=175317.78765461638, "Y"=530191.2650953768}, {"X"=175317.82558087553, "Y"=530191.3156396138}, {"X"=175317.86396142832, "Y"=530191.3661447766}, {"X"=175317.90213229894, "Y"=530191.4170345672}, {"X"=175317.94015622098, "Y"=530191.4673554361}, {"X"=175317.97785589864, "Y"=530191.5182610467}, {"X"=175318.0155045048, "Y"=530191.5692700257}, {"X"=175318.05364278206, "Y"=530191.620222066}, {"X"=175318.09153813362, "Y"=530191.6719994495}, {"X"=175318.1293183478, "Y"=530191.7246817079}, {"X"=175318.16774718426, "Y"=530191.7774419627}, {"X"=175318.20674981424, "Y"=530191.8298353782}, {"X"=175318.24521226567, "Y"=530191.8828796588}, 
